vi "1762AdiabaticPassageSequenceALLYBdouble.vi"(0 "Runs":dbl=500.0) -> ()   [LabVIEW 2009]
uses:
  <vilib>/Utility/file.llb/Write To Spreadsheet File (DBL).vi
panel:
  in  "second sweep freq":dbl=98.1
  out "deshelve attempts":dbl
  in  "Power (-12 Max)":dbl=-12.0
  in  "AP Sweep Width (MHz)":dbl=0.4
  in  "first sweep freq":dbl=98.1
  in  "Real Cutoff":i32=15
  in  "Sweep Duration (us)":dbl=500.0
  out "+/-":dbl=0.4472135954999579
  in  "Pump Expose Time (us)":dbl=3.0
  in  "Restart":bool
  out "Shelved Fraction":dbl=60.0
  out "Shelving Events":dbl=4.0
  out "Cut-off":i32=50
  out "Background":waveform(i32)(graph)={"t0"=timestamp(64.5 s since 1904-01-01), "dt"=1.0, "Y"=[1, 2, 1, 4, 2, 4, 2, 1, 3, 6, 4, 5, 6, 6, 5, 4, 6, 9, 5, 6, 10, 7, 5, 5, 9, 10, 2, 7, 8, 2, 6, 2, 10, 6, 3, 4, 2, 5, 2, 1, 2, 1, 1, 2, 2, 0, 0, 1, 1, 2]}
  out "+ / -":dbl=10.808259218610711
  out "Background":dbl=86.175
  in  "Interval":dbl=0.02
  out "Histogram":waveform(i32)(graph)={"t0"=timestamp(22.5 s since 1904-01-01), "dt"=1.0, "Y"=[1, 1, 1, 1, 0, 6, 2, 2, 3, 4, 7, 6, 5, 10, 5, 12, 9, 9, 11, 8, 6, 6, 14, 4, 7, 2, 1, 3, 3, 3, 1, 0, 1, 0, 3, 0, 0, 0, 0, 0, 0, 0, 0, 0, 0, 0, 0, 0, 0, 0, 0, 0, 0, 0, 0, 0, 0, 0, 0, 0, 0, 0, 0, 0, 0, 0, 0, 0, 0, 0, 0, 0, 0, 0, 0, 0, 0, 0, 0, 0, 0, 0, 1, 0, 0, 0, 0, 1, 0, 0, 1, 0, 2, 0, 1, 2, 0, 2, 0, 4, 5, 0, 0, 2, 3, 2, 3, 8, 4, 7, 6, 3, 7, 5, 6, 9, 6, 8, 4, 10, 4, 4, 7, 7, 6, 8, 11, 7, 12, 6, 13, 6, 7, 12, 11, 11, 2, 4, 5, 6, 7, 5, 5, 4, 5, 4, 3, 2, 4, 6, 3, 2, 3, 1, 0, 4, 2, 1, 2, 1, 2, 1, 2, 2, 1, 1, 1, 1, 0, 0, 1, 1, 1, 0, 0, 2, 0, 0, 2]}
  out "Run Number":dbl=6.0
  out "Path":path=path "c:/data/01-11-2009_14-34-35_0.1000001762AdiabaticPass.txt"
  out "Counts":i32=27
  out "Green":bool=TRUE
  out "Shelved?":bool=TRUE
  out "Red":bool=TRUE
  # "second sweep freq > first sweep\nsecond - first > sweep width"
  # "Interval"
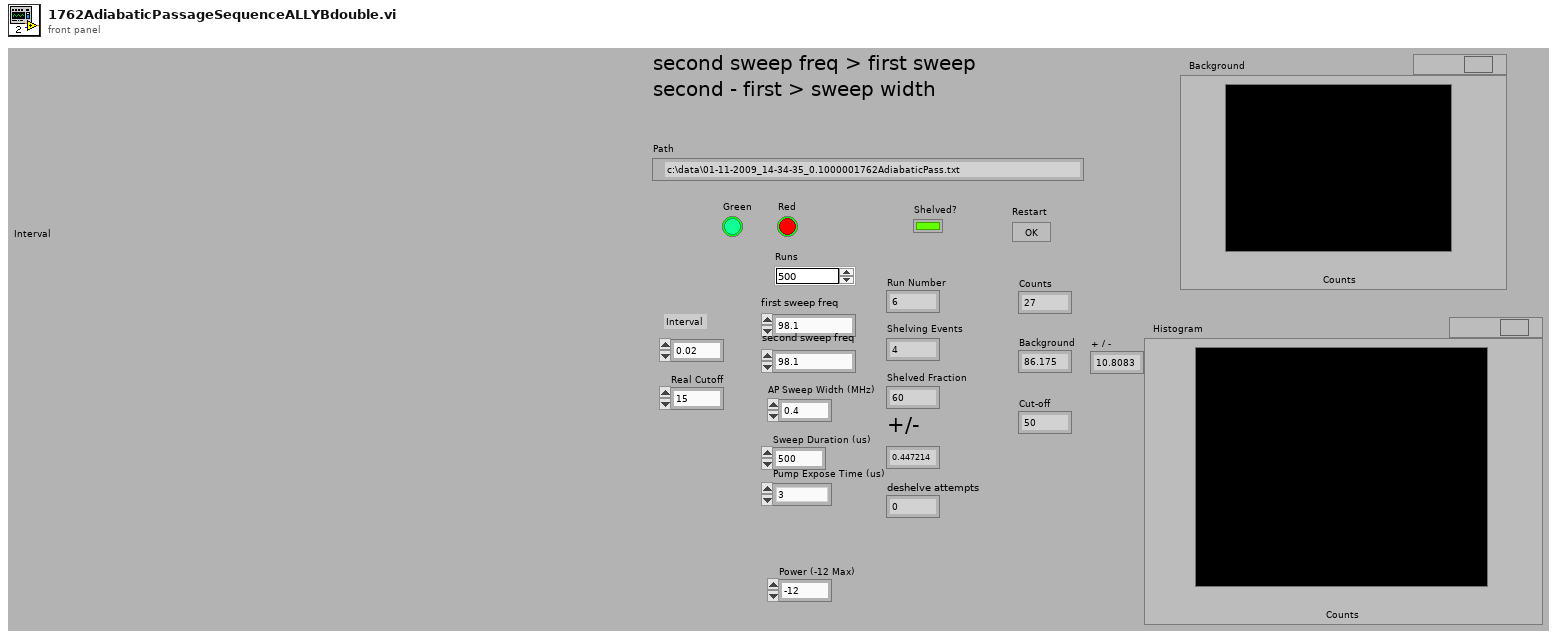
[diagram p1: front panel]
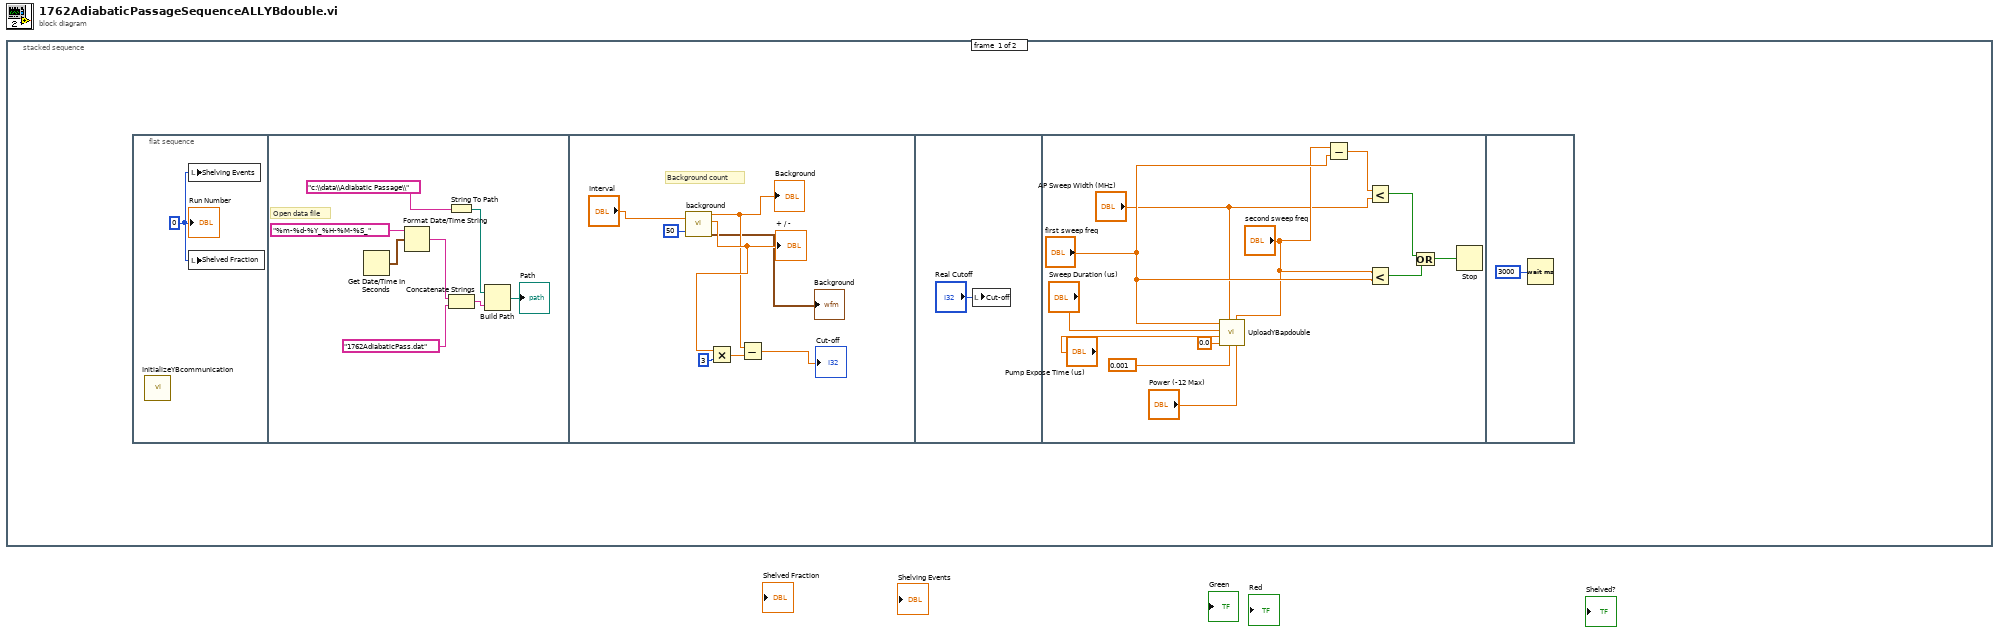
[diagram p0: block diagram]
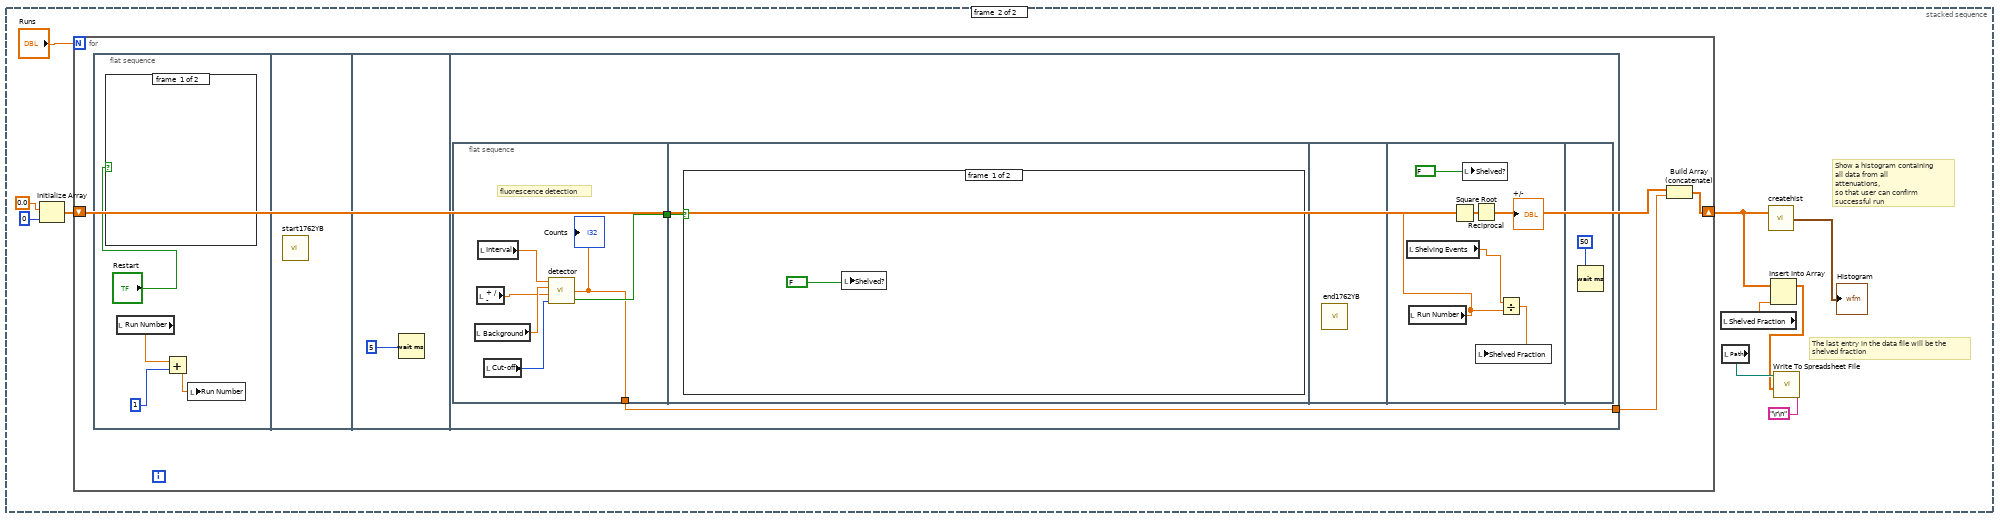
[diagram p2: hidden frame]
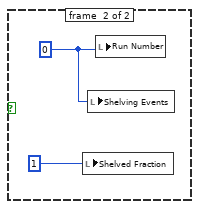
[diagram p3: hidden frame]
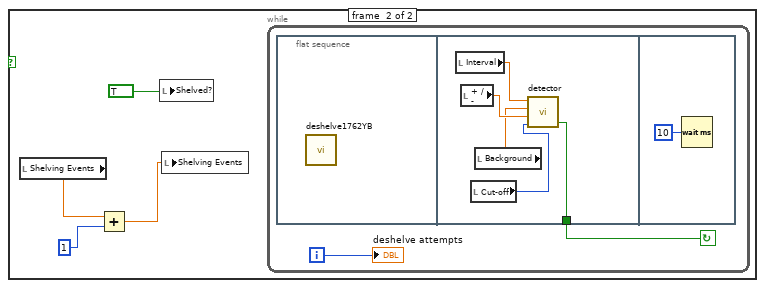
[diagram p4: hidden frame]
diagram:
  n1 = stacked-sequence {
    frame #0 {
      n2 = flat-sequence {
        frame #0 {
          w1 = 0
          n3 = call "InitializeYBcommunication.vi"() -> ()  [unwired: 12 in]
          n4 = local write "Shelving Events"(w1) -> ()
          n5 = local write "Shelved Fraction"(w1) -> ()
          "Run Number" <- w1
        }
        frame #1 {
          # "Open data file"
          n6 = Get Date/Time In Seconds() -> (seconds since 1Jan1904=w7:timestamp)
          n7 = Format Date/Time String(time format string (%c)="%m-%d-%Y_%H-%M-%S_", seconds (now)=w7) -> (date/time string=w9:string)  [unwired: 1 in]
          n8 = String To Path(string="c:\\data\\Adiabatic Passage\\") -> (path=w5:path)
          n9 = Concatenate Strings(w9, "1762AdiabaticPass.dat") -> (w3:string)
          n10 = Build Path(base path=w5, name or relative path=w3) -> (appended path=→"Path":path)
        }
        frame #2 {
          # "Background count"
          n11 = call "background.vi"("Interval"="Interval", "Runs"=50) -> ("Mean"=w14:dbl, "Deviation"=w17:dbl, "Histogram"=→"Background":waveform(i32))  [unwired: 1 out]
          "Background" <- w14
          "+ / -" <- w17
          n12 = Multiply(x=w17, y=3) -> (x*y=w15:dbl)
          n13 = Subtract(x=w14, y=w15) -> (x-y=→"Cut-off":dbl)
        }
        frame #3 {
          n14 = local write "Cut-off"("Real Cutoff") -> ()
        }
        frame #4 {
          n15 = call "UploadYBapdouble.vi"("Power"="Power (-12 Max)", "second sweep freq"="second sweep freq", "AP Freq Step"=0.001, "AP Sweep Width"="AP Sweep Width (MHz)", "RF time"=0.0, "OP Time"="Pump Expose Time (us)", "1762 Pulse Time"="Sweep Duration (us)", "first sweep freq"="first sweep freq") -> ()  [unwired: 4 in]
          n16 = Subtract(x="second sweep freq", y="first sweep freq") -> (x-y=w27:dbl)
          n17 = Less?(x=w27, y="AP Sweep Width (MHz)") -> (x < y?=w30:bool)
          n18 = Less?(x="second sweep freq", y="first sweep freq") -> (x < y?=w24:bool)
          n19 = Or(x=w30, y=w24) -> (x .or. y?=w25:bool)
          n20 = Stop(stop? (T)=w25) -> ()
        }
        frame #5 {
          n21 = Wait (ms)(milliseconds to wait=u32 3000) -> ()  [unwired: 1 out]
        }
      }
    }
    frame #1 {
      # "The last entry in the data file will be the\nshelved fraction"
      # "Show a histogram containing\nall data from all attenuations, \nso that user can confirm successful run"
      n22 = Initialize Array(0.0, 0) -> (w38:dbl[])
      n23 = for {
        N: "Runs" -> [_]
        shift-right: [w42] -> w35
        shift-left: w38 -> [w43]
        n24 = flat-sequence {
          tunnel: [w52] -> w44
          frame #0 {
            n25 = case shown="True" "Restart" {
              frame #0 {
              }
              frame #1 {
                w50 = 0
                n26 = local write "Shelved Fraction"(1) -> ()
                n27 = local write "Shelving Events"(w50) -> ()
                n28 = local write "Run Number"(w50) -> ()
              }
            }
            n29 = local read "Run Number"() -> (w47:dbl)
            n30 = Add(x=w47, y=1) -> (x+y=w46:dbl)
            n31 = local write "Run Number"(w46) -> ()
          }
          frame #1 {
            n32 = call "start1762YB.vi"() -> ()  [unwired: 11 in, 1 out]
          }
          frame #2 {
            n33 = Wait (ms)(milliseconds to wait=5) -> ()  [unwired: 1 out]
          }
          frame #3 {
            n34 = flat-sequence {
              tunnel: [w56] -> w53
              tunnel: [w55] -> w52
              tunnel: w53 -> [w60]
              frame #0 {
                # "fluorescence detection"
                n35 = local read "Background"() -> (w59:dbl)
                n36 = local read "+ / -"() -> (w58:dbl)
                n37 = local read "Interval"() -> (w57:dbl)
                n38 = local read "Cut-off"() -> (w54:i32)
                n39 = call "detector.vi"("Cutoff"=w54, "+ / -"=w58, "Background"=w59, "Interval"=w57) -> ("Boolean"=w56:bool, "Counts"=w55:dbl)  [unwired: 1 in]
                "Counts" <- w55
              }
              frame #1 {
                n40 = case shown="True" w60 {
                  frame #0 {
                    n41 = local write "Shelved?"(FALSE) -> ()
                  }
                  frame #1 {
                    n42 = local read "Shelving Events"() -> (w64:dbl)
                    n43 = Add(x=w64, y=1) -> (x+y=w63:dbl)
                    n44 = local write "Shelved?"(TRUE) -> ()
                    n45 = local write "Shelving Events"(w63) -> ()
                    n46 = while {
                      i -> [w66]
                      stop <- w67 continue-if-true
                      n47 = flat-sequence {
                        tunnel: [w72] -> w67
                        frame #0 {
                          n48 = call "deshelve1762YB.vi"() -> ()  [unwired: 11 in, 1 out]
                        }
                        frame #1 {
                          n49 = local read "Interval"() -> (w69:dbl)
                          n50 = local read "+ / -"() -> (w71:dbl)
                          n51 = local read "Cut-off"() -> (w68:i32)
                          n52 = local read "Background"() -> (w70:dbl)
                          n53 = call "detector.vi"("Cutoff"=w68, "+ / -"=w71, "Background"=w70, "Interval"=w69) -> ("Boolean"=w72:bool)  [unwired: 1 in, 1 out]
                        }
                        frame #2 {
                          n54 = Wait (ms)(milliseconds to wait=u32 10) -> ()  [unwired: 1 out]
                        }
                      }
                      "deshelve attempts" <- w66
                    }
                  }
                }
              }
              frame #2 {
                n55 = call "end1762YB.vi"() -> ()  [unwired: 1 in]
              }
              frame #3 {
                n56 = local read "Shelving Events"() -> (w79:dbl)
                n57 = local read "Run Number"() -> (w75:dbl)
                n58 = Square Root(x=w75) -> (sqrt(x)=w77:dbl)
                n59 = local write "Shelved?"(FALSE) -> ()
                n60 = Reciprocal(x=w77) -> (1/x=→"+/-":dbl)
                n61 = Divide(x=w79, y=w75) -> (x/y=w74:dbl)
                n62 = local write "Shelved Fraction"(w74) -> ()
              }
              frame #4 {
                n63 = Wait (ms)(milliseconds to wait=u32 50) -> ()  [unwired: 1 out]
              }
            }
          }
        }
        n64 = Build Array (concatenate)(w43, w44) -> (w42:dbl[])
      }
      n65 = local read "Shelved Fraction"() -> (w34:dbl)
      n66 = local read "Path"() -> (w41:path)
      n67 = call "createhist.vi"("Array"=w35) -> ("Waveform Graph"=→"Histogram":waveform(i32))  [unwired: 1 in]
      n68 = Insert Into Array(array=w35, new element=w34) -> (w33:dbl[])  [unwired: 1 in]
      n69 = call-poly <vilib>:"Write To Spreadsheet File.vi"("delimiter (\\t)"="\r\n", "1D data"=w33, "file path (dialog if empty)"=w41) -> ()  [unwired: 5 in, 1 out]
    }
  }
